vi "Read FK Table.vi"(8 "error in (no error)":errorcluster, 11 "FK Ring in":refnum<class "FK Ring.lvclass">) -> (0 "error out":errorcluster, 2 "PK Table":string, 3 "FK Ring out":refnum<class "FK Ring.lvclass">)   [LabVIEW 2020, in "Old Basic Fields.lvlib" / "FK Ring.lvclass"]
uses:
  FK Ring.lvclass
  FK Ring.lvclass/FK Ring.ctl
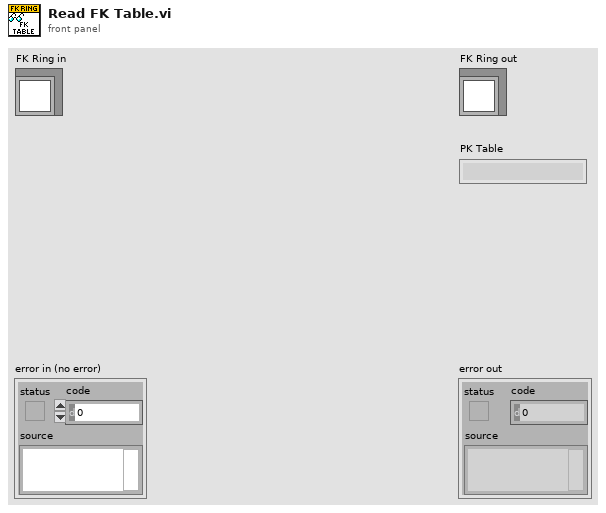
[diagram p1: front panel]
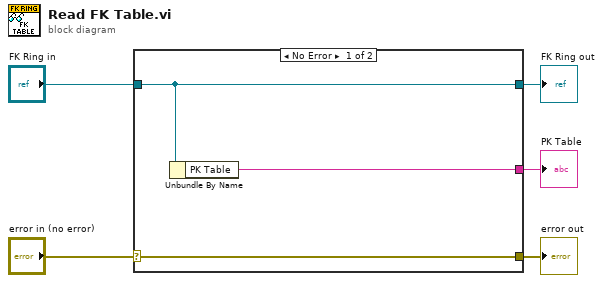
[diagram p0: block diagram]
diagram:
  n1 = case shown="No Error" "error in (no error)" {
    selector: "error in (no error)" -> [w8 w9]
    tunnel: [w8 w9] -> w4
    tunnel: [w7 w10] -> w2
    tunnel: "FK Ring in" -> [w7 w10]
    tunnel: [w6 _] -> w1
    frame No Error {
      n2 = Unbundle By Name(w7) -> ("PK Table"=w6:string)
    }
    frame Error {
    }
  }
  "error out" <- w4
  "FK Ring out" <- w2
  "PK Table" <- w1
